vi "cw7_d.vi"() -> ()   [LabVIEW 2012]
panel:
  out "Posortowana":bool
  out "Posortowana tablica":dbl[](array[numeric])
  in  "Array":dbl[](array[numeric])
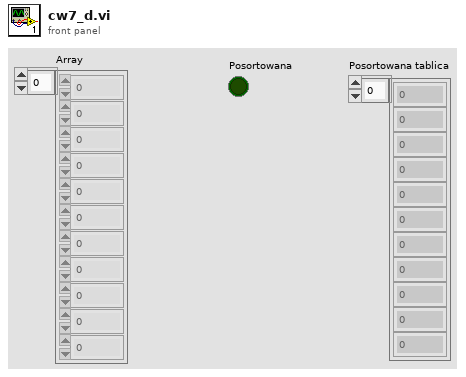
[diagram p1: front panel]
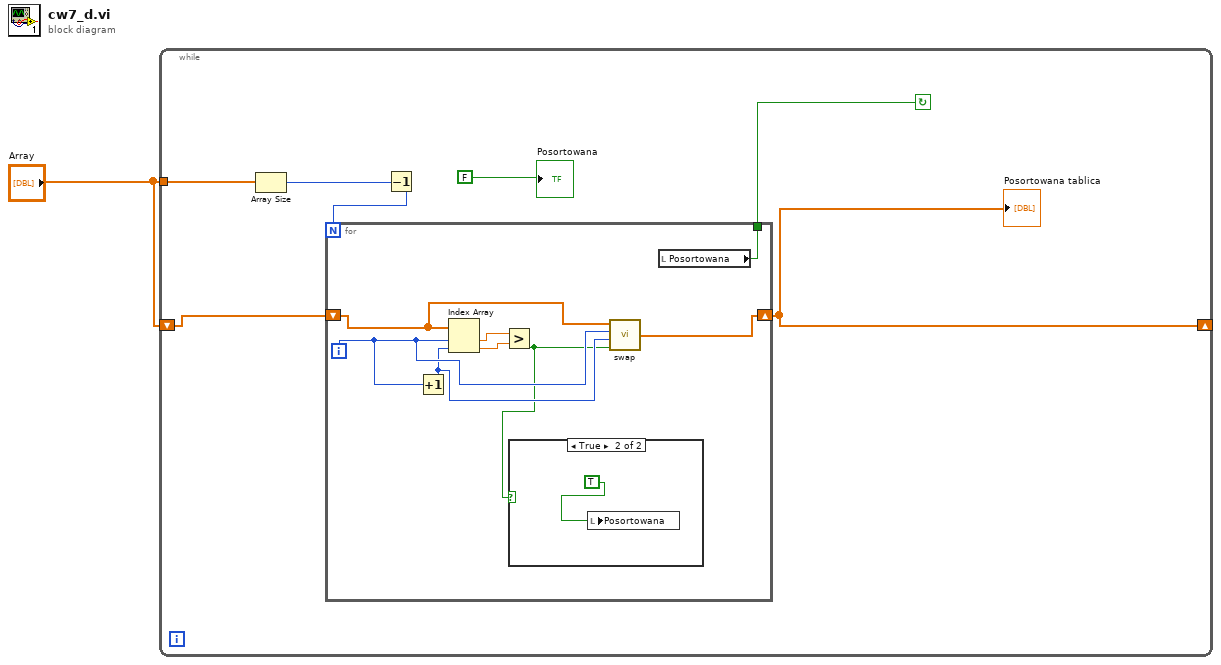
[diagram p0: block diagram]
diagram:
  n1 = while {
    tunnel: "Array" -> [w6]
    shift-right: [w3] -> _
    shift-left: "Array" -> [w4]
    stop <- w2 continue-if-true
    n2 = Array Size(array=w6) -> (size(s)=w8:i32)
    n3 = Decrement(x=w8) -> (x-1=w7:i32)
    n4 = for {
      N: w7 -> [_]
      shift-right: [w11] -> w3
      shift-left: w4 -> [w12]
      tunnel: [w9] -> w2
      i -> [w14]
      n5 = Increment(x=w14) -> (x+1=w13:i32)
      n6 = Index Array(array=w12, index #1=w14, index #2=w13) -> (element #1=w16:dbl, element #2=w15:dbl)
      n7 = Greater?(x=w16, y=w15) -> (0:w10:bool)
      n8 = case shown="True" w10 {
        frame False {
        }
        frame True {
          n9 = local write "Posortowana"(TRUE) -> ()
        }
      }
      n10 = call "swap.vi"("Swap"=w10, "index 2"=w13, "index 1"=w14, "Array"=w12) -> ("Swapped Array"=w11:dbl[])
      n11 = local read "Posortowana"() -> (w9:bool)
    }
    "Posortowana tablica" <- w3
    "Posortowana" <- FALSE
  }
